vi "源强与基线.vi"(1 "通量in":dbl[](array[numeric]), 7 "通量名称：":string[](array[string]), 8 "执行:调用时显示前面板":bool, 9 "记忆本底":dbl[](array[numeric]), 10 "记忆源强":dbl[](array[numeric])) -> (0 "源与基线灯":bool, 2 "面板开":bool, 3 "通量out":dbl[](array[numeric]), 4 "改动本底":dbl[](array[numeric]), 5 "源强out":dbl[](array[numeric]))   [LabVIEW 2020]
panel:
  in  "本底减除：":dbl[](array[numeric])
  in  "通道源强：":dbl[](array[numeric])
  in  "源与本底开关：":bool
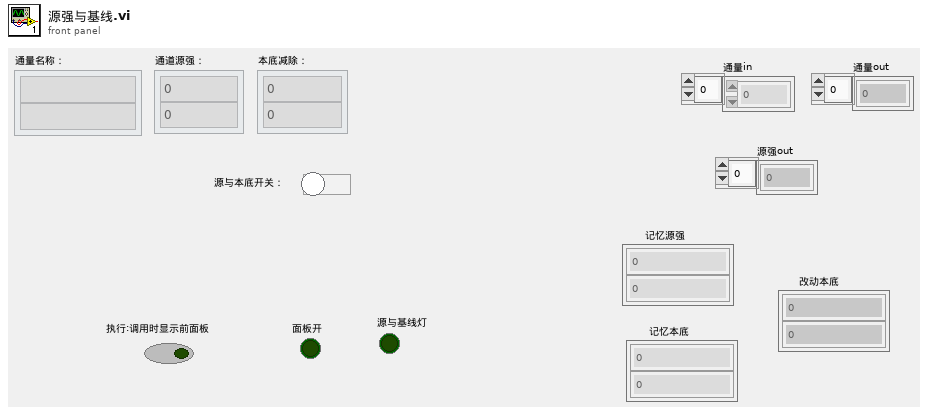
[diagram p1: front panel]
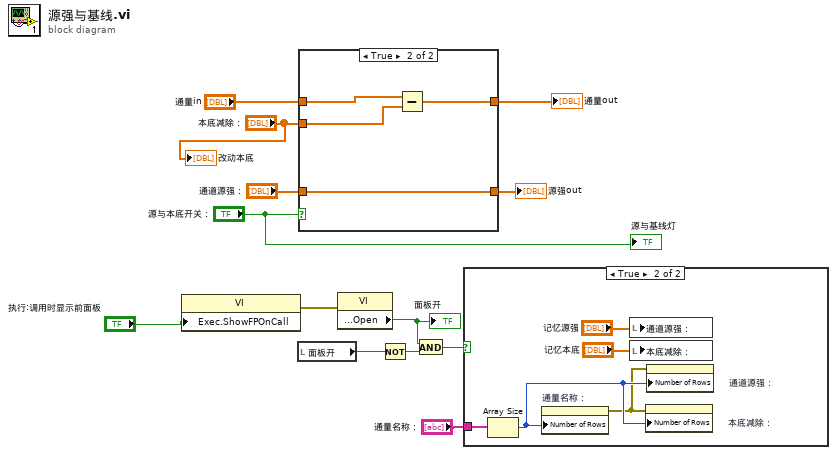
[diagram p0: block diagram]
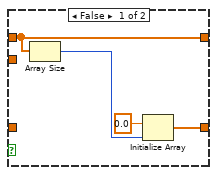
[diagram p3: hidden frame]
diagram:
  n1 = property class="VI"("Exec.ShowFPOnCall"="执行:调用时显示前面板") -> (error out=w11:errorcluster)  [unwired: 2 in, 1 out]
  n2 = local read "面板开"() -> (w10:bool)
  n3 = case shown="True" "源与本底开关：" {
    tunnel: "通量in" -> [w15 w20]
    tunnel: [w15 w19] -> w1
    tunnel: "通道源强：" -> [_ w21]
    tunnel: "本底减除：" -> [_ w18]
    tunnel: [w16 w21] -> w4
    frame False {
      n4 = Array Size(array=w15) -> (size(s)=w14:i32)
      n5 = Initialize Array(0.0 ("元素"), w14) -> (w16:dbl[])
    }
    frame True {
      n6 = Subtract(x=w20, y=w18) -> (x-y=w19:dbl[])
    }
  }
  "通量out" <- w1
  "源强out" <- w4
  n7 = property class="VI"(error in=w11) -> ("Front Panel.Open"=w8:bool)  [unwired: 1 in, 2 out]
  "面板开" <- w8
  n8 = Not(x=w10) -> (.not. x?=w9:bool)
  n9 = And(x=w8, y=w9) -> (x .and. y?=w7:bool)
  n10 = case shown="True" w7 {
    tunnel: "通量名称：" -> [_ w26]
    frame False {
    }
    frame True {
      n11 = Array Size(array=w26) -> (size(s)=w25:i32)
      n12 = property on="通量名称：" class="Arr (strict)"("Number of Rows"=w25) -> (error out=w24:errorcluster)  [unwired: 2 in, 1 out]
      n13 = local write "通道源强："("记忆源强") -> ()
      n14 = local write "本底减除："("记忆本底") -> ()
      n15 = property on="本底减除：" class="Arr (strict)"(error in=w24, "Number of Rows"=w25) -> ()  [unwired: 1 in, 2 out]
      n16 = property on="通道源强：" class="Arr (strict)"(error in=w24, "Number of Rows"=w25) -> ()  [unwired: 1 in, 2 out]
    }
  }
  "源与基线灯" <- "源与本底开关："
  "改动本底" <- "本底减除："
